vi "write_png.vi"() -> ()   [LabVIEW 2019]
panel:
  in  "Create All":bool
  out "Structures Path":path
  in  "Stop":bool
  in  "Create":bool
  in  "VI Path":path
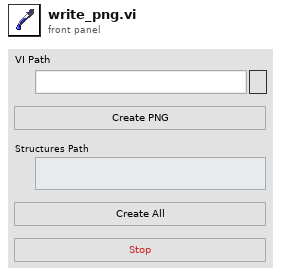
[diagram p1: front panel]
types:
  T1 = typedef "imagedata.ctl" = cluster{"image type":i32, "image depth":i32, "image":u8[], "mask":u8[], "colors":u32[], "Rectangle":cluster{"left":i16, "top":i16, "right":i16, "bottom":i16}}
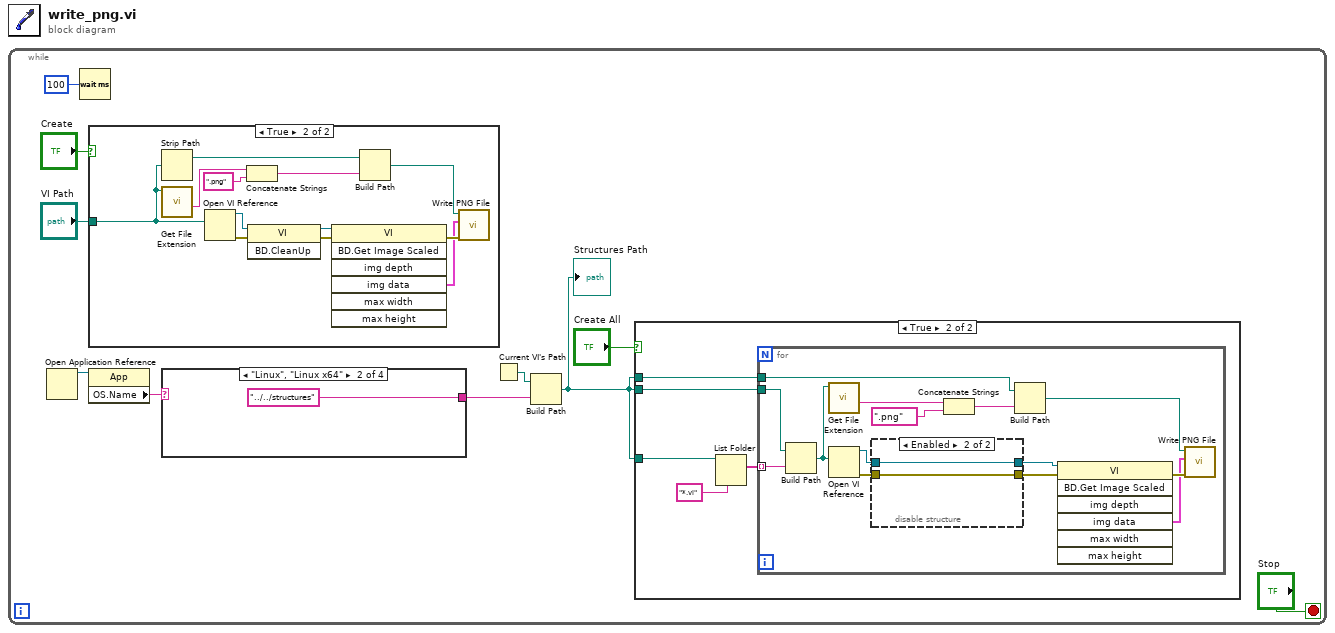
[diagram p0: block diagram]
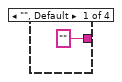
[diagram p2: hidden frame]
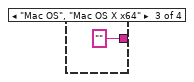
[diagram p3: hidden frame]
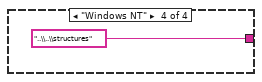
[diagram p4: hidden frame]
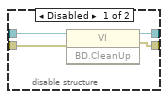
[diagram p6: hidden frame]
diagram:
  n1 = while {
    stop <- "Stop" stop-if-true
    n2 = Open Application Reference() -> (3:w5:refnum<vi>)  [unwired: 4 in, 1 out]
    n3 = Wait (ms)(milliseconds to wait=u32 100) -> ()  [unwired: 1 out]
    n4 = case shown="True" "Create" {
      tunnel: "VI Path" -> [_ w45]
      frame False {
      }
      frame True {
        n5 = Strip Path(path=w45) -> (stripped path=w44:path)  [unwired: 1 out]
        n6 = call <vilib>:"Get File Extension.vi"("file"=w45) -> ("filename without extension"=w41:string)  [unwired: 6 in, 4 out]
        n7 = Open VI Reference(vi path=w45) -> (vi reference=w51:refnum<vi>, error out=w48:errorcluster)  [unwired: 5 in]
        n8 = Concatenate Strings(w41, ".png" ("string")) -> (w40:string)
        n9 = invoke class="VI" method="BD.CleanUp"(reference=w51, error in=w48) -> (reference out=w50:refnum<vi>, error out=w49:errorcluster)  [unwired: 1 in, 1 out]
        n10 = invoke class="VI" method="BD.Get Image Scaled"(reference=w50, error in=w49) -> (error out=w47:errorcluster, "img data"=w46:T1)  [unwired: 5 in, 5 out]
        n11 = Build Path(base path=w44, name or relative path=w40) -> (appended path=w43:path)
        n12 = call <vilib>:"Write PNG File.vi"("error in (no error)"=w47, "image data"=w46, "path to PNG file"=w43) -> ()  [unwired: 7 in, 2 out]
      }
    }
    n13 = property class="App"(reference=w5) -> ("OS.Name"=w4:string)  [unwired: 1 in, 2 out]
    n14 = case shown="\"Linux\", \"Linux x64\"" w4 {
      tunnel: ["" ("return type") "../../structures" ("name or relative path") "" ("return type") "..\\..\\structures" ("name or relative path")] -> w2
      frame "", Default {
      }
      frame "Linux", "Linux x64" {
      }
      frame "Mac OS", "Mac OS X x64" {
      }
      frame "Windows NT" {
      }
    }
    n15 = Current VI's Path() -> (path=w3:path)
    n16 = Build Path(base path=w3, name or relative path=w2) -> (appended path=w1:path)
    "Structures Path" <- w1
    n17 = case shown="True" "Create All" {
      tunnel: w1 -> [_ w17]
      tunnel: w1 -> [_ w16]
      tunnel: w1 -> [_ w15]
      frame False {
      }
      frame True {
        n18 = List Folder(path=w15, pattern="*.vi") -> (filenames=w18:string[])  [unwired: 2 in, 3 out]
        n19 = for {
          tunnel: w18 -> [w33] mode=indexing
          tunnel: w17 -> [w22]
          tunnel: w16 -> [w21]
          n20 = Build Path(base path=w22, name or relative path=w33) -> (appended path=w27:path)
          n21 = call <vilib>:"Get File Extension.vi"("file"=w27) -> ("filename without extension"=w25:string)  [unwired: 6 in, 4 out]
          n22 = Open VI Reference(vi path=w27) -> (vi reference=w28:refnum<vi>, error out=w20:errorcluster)  [unwired: 5 in]
          n23 = disable-structure shown="Enabled" {
            disable-tunnel: [w37 w39] -> w32
            disable-tunnel: [w36 w38] -> w31
            disable-tunnel: w28 -> [w35 w39]
            disable-tunnel: w20 -> [w34 w38]
            frame Disabled {
              n24 = invoke class="VI" method="BD.CleanUp"(reference=w35, error in=w34) -> (reference out=w37:refnum<vi>, error out=w36:errorcluster)  [unwired: 1 in, 1 out]
            }
            frame Enabled {
            }
          }
          n25 = Concatenate Strings(w25, ".png" ("string")) -> (w24:string)
          n26 = Build Path(base path=w21, name or relative path=w24) -> (appended path=w23:path)
          n27 = invoke class="VI" method="BD.Get Image Scaled"(reference=w32, error in=w31) -> (error out=w30:errorcluster, "img data"=w29:T1)  [unwired: 5 in, 5 out]
          n28 = call <vilib>:"Write PNG File.vi"("error in (no error)"=w30, "image data"=w29, "path to PNG file"=w23) -> ()  [unwired: 7 in, 2 out]
        }
      }
    }
  }
